vi "Entry.vi"(8 "error in (no error)":errorcluster, 10 "Context in":refnum<class "Context.lvclass">, 11 "Logging in":refnum<class "Logging.lvclass">) -> (0 "error out":errorcluster, 2 "Context out":refnum<class "Context.lvclass">, 3 "Logging out":refnum<class "Logging.lvclass">)   [LabVIEW 2024, in "State.lvlib" / "Logging.lvclass"]
uses:
  Logging.lvclass
  Logging.lvclass/Logging.ctl
  Context/Context/Context.lvclass
panel:
  # "ENTRY TO LOGGING!"
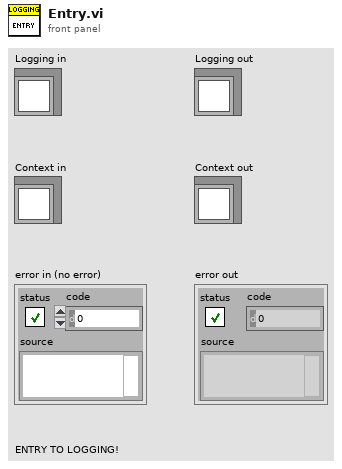
[diagram p1: front panel]
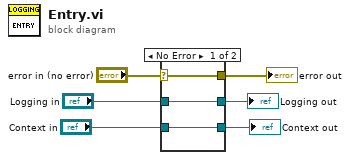
[diagram p0: block diagram]
diagram:
  n1 = case shown="No Error" "error in (no error)" {
    selector: "error in (no error)" -> [w9 w12]
    tunnel: [w9 w12] -> w6
    tunnel: "Context in" -> [w8 w11]
    tunnel: [w8 w11] -> w5
    tunnel: [w7 w10] -> w4
    tunnel: "Logging in" -> [w7 w10]
    frame No Error {
    }
    frame Error {
    }
  }
  "error out" <- w6
  "Logging out" <- w4
  "Context out" <- w5
